vi "FireLauncher.vi"   [LabVIEW 2013]
uses:
  <vilib>/Rock Robotics/WPI/Solenoid/WPI_SolenoidValue.ctl
  <vilib>/Rock Robotics/WPI/Solenoid/WPI_SolenoidSetEnum.vi
  Robot Global Data.vi
types:
  T1 = typedef "WPI_SolenoidValue.ctl" = enum16{"Off", "On", "Forward", "Reverse"}
  T2 = typedef "WPI_SolenoidDevRef.ctl" = cluster{"DevStatus":errorcluster, "Solenoid Module":T3, "Forward Solenoid Channel":T4, "Reverse Solenoid Channel":T4}
  T3 = typedef "FPGA_TypedefSolenoidModule.ctl" = enum16{"Solenoid Module 1", "Solenoid Module 2"}
  T4 = typedef "WPI_SolenoidChannel.ctl" = enum8{"Solenoid 1", "Solenoid 2", "Solenoid 3", "Solenoid 4", "Solenoid 5", "Solenoid 6", "Solenoid 7", "Solenoid 8", "Invalid"}
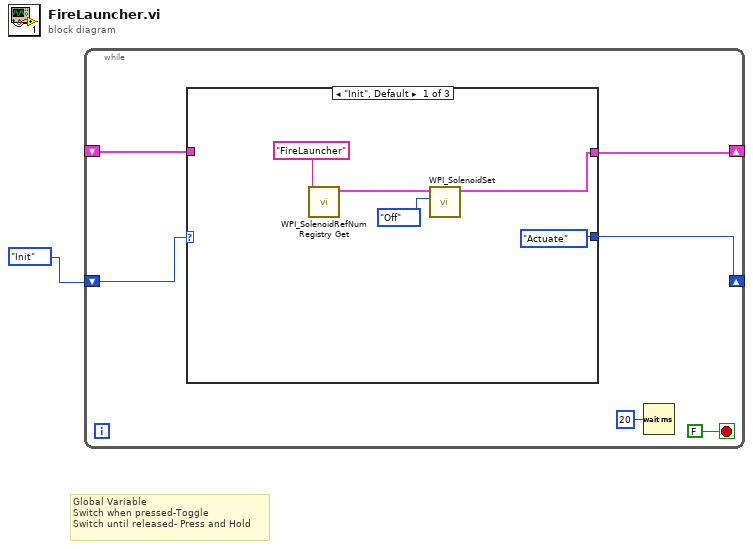
[diagram p0: block diagram]
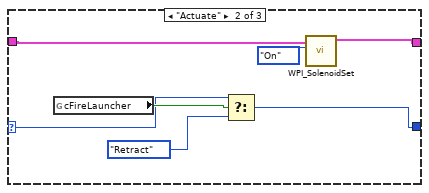
[diagram p2: hidden frame]
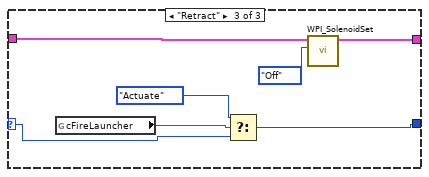
[diagram p3: hidden frame]
diagram:
  # "Global Variable\nSwitch when pressed-Toggle\nSwitch until released- Press and Hold"
  n1 = while {
    shift-right: [w6] -> _
    shift-left: enum16{"Init", "Actuate", "Retract"}."Init" -> [w7]
    shift-right: [w5] -> _
    shift-left: _ -> [w4]
    stop <- FALSE stop-if-true
    n2 = case shown="\"Init\", Default" w7 {
      selector: w7 -> [_ w13 w20]
      tunnel: [enum16{"Init", "Actuate", "Retract"}."Actuate" w15 w21] -> w6
      tunnel: [w9 w19 w23] -> w5
      tunnel: w4 -> [_ w18 w24]
      frame "Init", Default {
        n3 = call <vilib>:"WPI_SolenoidRefNum Registry Get.vi"("refnum name"="FireLauncher") -> ("SolenoidDevRef"=w10:T2)  [unwired: 9 in, 1 out]
        n4 = call-poly <vilib>:"WPI_SolenoidSet.vi"("Value"=WPI_SolenoidValue."Off", "SolenoidDevRef"=w10) -> ("SolenoidDevRef"=w9:T2)  [unwired: 8 in, 1 out]
      }
      frame "Actuate" {
        n5 = global read "Robot Global Data.vi" "cFireLauncher"() -> (w17:bool)
        n6 = Select(t=w13, s=w17, f=enum16{"Init", "Actuate", "Retract"}."Retract") -> (s? t:f=w15:enum16{"Init", "Actuate", "Retract"})
        n7 = call-poly <vilib>:"WPI_SolenoidSet.vi"("Value"=WPI_SolenoidValue."On", "SolenoidDevRef"=w18) -> ("SolenoidDevRef"=w19:T2)  [unwired: 8 in, 1 out]
      }
      frame "Retract" {
        n8 = global read "Robot Global Data.vi" "cFireLauncher"() -> (w26:bool)
        n9 = Select(t=enum16{"Init", "Actuate", "Retract"}."Actuate", s=w26, f=w20) -> (s? t:f=w21:enum16{"Init", "Actuate", "Retract"})
        n10 = call-poly <vilib>:"WPI_SolenoidSet.vi"("Value"=WPI_SolenoidValue."Off", "SolenoidDevRef"=w24) -> ("SolenoidDevRef"=w23:T2)  [unwired: 8 in, 1 out]
      }
    }
    n11 = Wait (ms)(milliseconds to wait=u32 20) -> ()  [unwired: 1 out]
  }
